vi "DAQ_Initialization_2.vi"(4 "AO Lasers":tag="USB-6363/ao0:3", 5 "AO Z":tag="USB-6211/ao1", 6 "AO Pockels":tag="USB-6211/ao0", 7 "DO":tag="USB-6363/port0/line0:4", 8 "error in (no error)":errorcluster, 9 "Counter":tag="USB-6363/ctr0") -> (0 "error out":errorcluster)   [LabVIEW 2025]
uses:
  <vilib>/DAQmx/create/channels.llb/DAQmx Create Channel (AO-Voltage-Basic).vi
  <vilib>/DAQmx/create/channels.llb/DAQmx Create Channel (DO-Digital Output).vi
  <vilib>/DAQmx/configure/timing.llb/DAQmx Timing (Sample Clock).vi
  <vilib>/DAQmx/configure/trigger.llb/DAQmx Start Trigger (Digital Edge).vi
  <vilib>/DAQmx/create/channels.llb/DAQmx Create Channel (CO-Pulse Generation-Time).vi
  <resource>/objmgr/daqmx.rc
  <vilib>/DAQmx/configure/events/hardwareSignals.llb/DAQmx Export Signal (Most Signals).vi
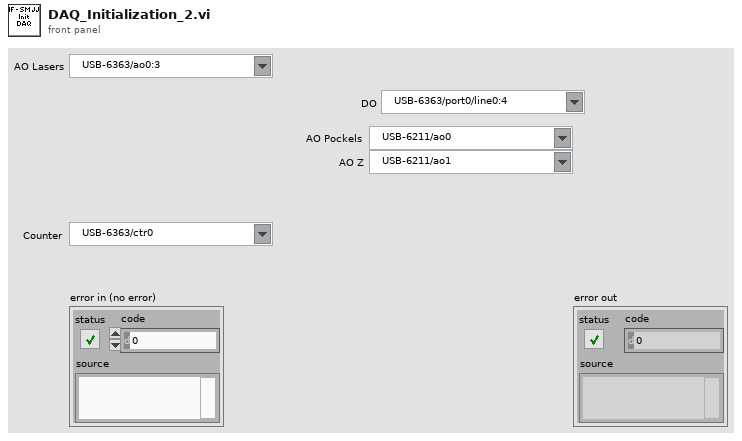
[diagram p1: front panel]
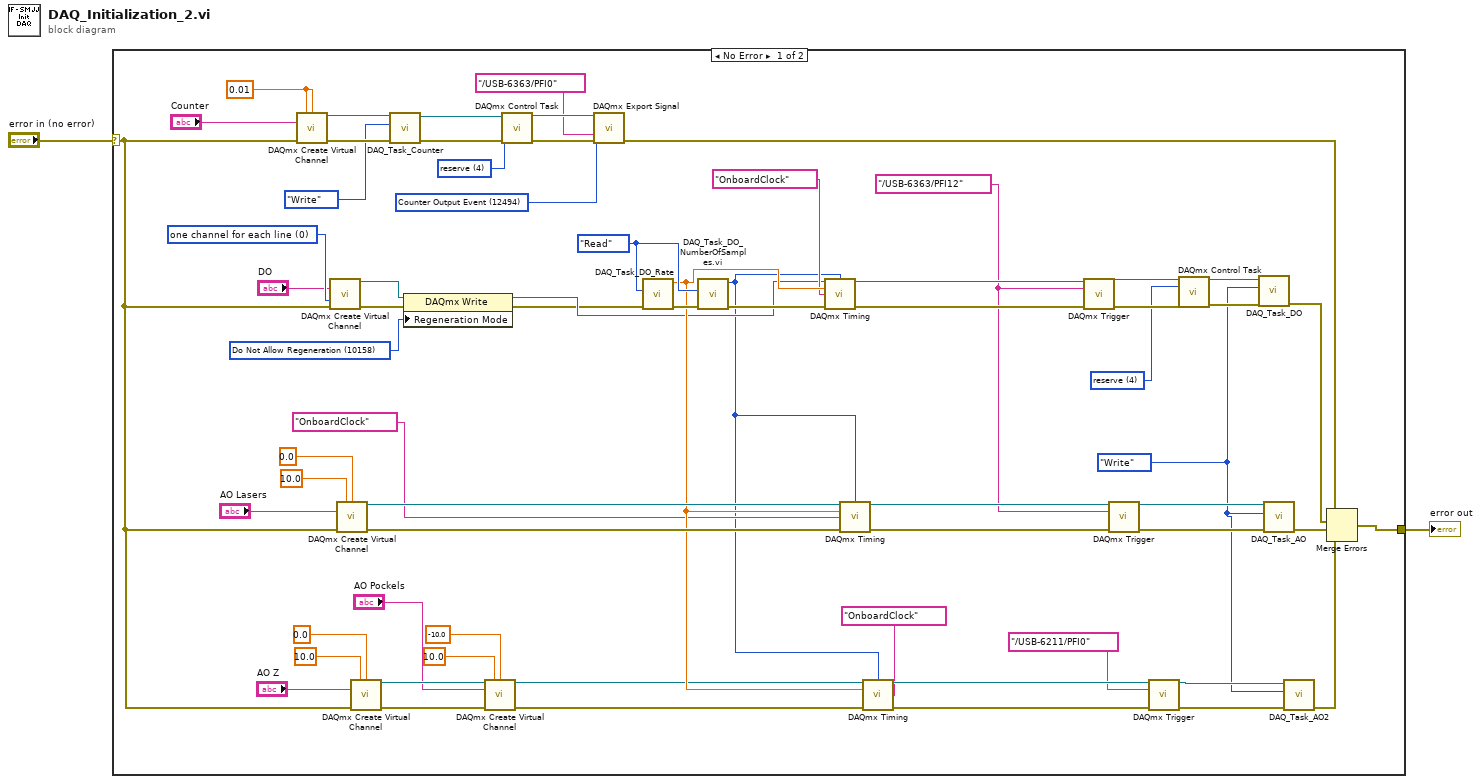
[diagram p0: block diagram]
diagram:
  n1 = case shown="No Error" "error in (no error)" {
    selector: "error in (no error)" -> [w11 w69]
    tunnel: [w12 w69] -> w1
    frame No Error {
      w4 = 12494 items=["AI Convert Clock"=12484, "10MHz Reference Clock"=12536, "20MHz Timebase Clock"=12486, "Sample Clock"=12487, "Advance Trigger"=12488, "Reference Trigger"=12490, "Start Trigger"=12491, "Advance Complete Event"=12492, "AI Hold Complete Event"=12493, "Counter Output Event"=12494, "Change Detection Event"=12511, "Watchdog Timer Expired Event"=12512] ("signal")
      w16 = enum16{"Write", "Read"}."Write" ("Action")
      w9 = tag "/USB-6363/PFI12" ("Timing source")
      w22 = 4 items=["verify"=2, "reserve"=4, "commit"=3, "unreserve"=5, "abort"=6] ("action")
      w28 = 4 items=["verify"=2, "reserve"=4, "commit"=3, "unreserve"=5, "abort"=6] ("action")
      w68 = 0 items=["one channel for each line", "one channel for all lines"] ("line grouping")
      w67 = enum16{"Write", "Read"}."Read" ("Action")
      w62 = 10158 items=["Allow Regeneration"=10097, "Do Not Allow Regeneration"=10158] ("RegenMode")
      w61 = 0.01 ("low time")
      n2 = call-poly <vilib>:"DAQmx Create Virtual Channel.vi"("high time"=w61, "low time"=w61, "counter"="Counter", "error in"=w11) -> ("task out"=w32:refnum<k21>, "error out"=w31:errorcluster)  [unwired: 10 in]
      n3 = call-poly <vilib>:"DAQmx Create Virtual Channel.vi"("lines"="DO", "line grouping"=w68, "error in"=w11) -> ("task out"=w64:refnum<k21>, "error out"=w63:errorcluster)  [unwired: 11 in]
      n4 = call-poly <vilib>:"DAQmx Create Virtual Channel.vi"("maximum value"=10.0, "minimum value"=0.0, "physical channels"="AO Lasers", "error in"=w11) -> ("task out"=w55:refnum<k21>, "error out"=w54:errorcluster)  [unwired: 10 in]
      n5 = call-poly <vilib>:"DAQmx Create Virtual Channel.vi"("maximum value"=10.0, "minimum value"=0.0, "physical channels"="AO Z", "error in"=w11) -> ("task out"=w42:refnum<k21>, "error out"=w43:errorcluster)  [unwired: 10 in]
      n6 = call "DAQ_Task_Counter.vi"("error in"=w31, "Action"=enum16{"Write", "Read"}."Write", "DAQ_Task_Counter"=w32) -> ("error out"=w29:errorcluster, "DAQ_Task_Counter"=w30:refnum<k21>)  [unwired: 7 in]
      n7 = property class="DAQmx Write"(reference=w64, error in=w63, "Regeneration Mode"=w62) -> (reference out=w26:refnum<k21>, error out=w25:errorcluster)
      n8 = call-poly <vilib>:"DAQmx Create Virtual Channel.vi"("task in"=w42, "maximum value"=10.0, "minimum value"=-10.0, "physical channels"="AO Pockels", "error in"=w43) -> ("task out"=w40:refnum<k21>, "error out"=w39:errorcluster)  [unwired: 9 in]
      n9 = call <vilib>:"DAQmx Control Task.vi"("task/channels in"=w30, "action"=w28, "error in"=w29) -> ("task out"=w7:refnum<k21>, "error out"=w6:errorcluster)  [unwired: 11 in]
      n10 = call-poly <vilib>:"DAQmx Export Signal.vi"("task/channels in"=w7, "signal"=w4, "output terminal"=tag "/USB-6363/PFI0", "error in"=w6) -> ("error out"=w5:errorcluster)  [unwired: 10 in, 1 out]
      n11 = call "DAQ_Task_DO_Rate.vi"("error in"=w25, "Action"=w67) -> ("error out"=w65:errorcluster, "DO_Rate"=w45:dbl)  [unwired: 8 in]
      n12 = call "DAQ_Task_DO_NumberOfSamples.vi.vi"("error in"=w65, "Action"=w67) -> ("error out"=w66:errorcluster, "Samples"=w10:u32)  [unwired: 8 in]
      n13 = call-poly <vilib>:"DAQmx Timing.vi"("task/channels in"=w26, "samples per channel"=w10, "rate"=w45, "source"=tag "OnboardClock", "error in"=w66) -> ("task out"=w18:refnum<k21>, "error out"=w19:errorcluster)  [unwired: 9 in]
      n14 = call-poly <vilib>:"DAQmx Timing.vi"("task/channels in"=w55, "samples per channel"=w10, "rate"=w45, "source"=tag "OnboardClock", "error in"=w54) -> ("task out"=w34:refnum<k21>, "error out"=w48:errorcluster)  [unwired: 9 in]
      n15 = call-poly <vilib>:"DAQmx Timing.vi"("task/channels in"=w40, "samples per channel"=w10, "rate"=w45, "source"=tag "OnboardClock", "error in"=w39) -> ("task out"=w46:refnum<k21>, "error out"=w47:errorcluster)  [unwired: 9 in]
      n16 = call-poly <vilib>:"DAQmx Trigger.vi"("task/channels in"=w18, "source"=w9, "error in"=w19) -> ("task out"=w23:refnum<k21>, "error out"=w24:errorcluster)  [unwired: 11 in]
      n17 = call-poly <vilib>:"DAQmx Trigger.vi"("task/channels in"=w34, "source"=w9, "error in"=w48) -> ("task out"=w53:refnum<k21>, "error out"=w52:errorcluster)  [unwired: 11 in]
      n18 = call-poly <vilib>:"DAQmx Trigger.vi"("task/channels in"=w46, "source"=tag "/USB-6211/PFI0", "error in"=w47) -> ("task out"=w36:refnum<k21>, "error out"=w44:errorcluster)  [unwired: 11 in]
      n19 = call <vilib>:"DAQmx Control Task.vi"("task/channels in"=w23, "action"=w22, "error in"=w24) -> ("task out"=w21:refnum<k21>, "error out"=w20:errorcluster)  [unwired: 11 in]
      n20 = call "DAQ_Task_DO.vi"("error in"=w20, "Action"=w16, "DAQ_Task_DO"=w21) -> ("error out"=w15:errorcluster)  [unwired: 7 in, 1 out]
      n21 = call "DAQ_Task_AO.vi"("error in"=w52, "Action"=w16, "DAQ_Task_AO"=w53) -> ("error out"=w14:errorcluster)  [unwired: 7 in, 1 out]
      n22 = call "DAQ_Task_AO2.vi"("error in"=w44, "Action"=w16, "DAQ_Task_AO2"=w36) -> ("error out"=w13:errorcluster)  [unwired: 7 in, 1 out]
      n23 = Merge Errors(w5, w15, w14, w13) -> (w12:errorcluster)
    }
    frame Error {
    }
  }
  "error out" <- w1
